vi "Assert Not Error 1097.vi"(8 "error in (no error)":errorcluster, 11 "actual value":errorcluster) -> (0 "error out":errorcluster)   [LabVIEW 2013, in "libssh2_tests.lvlib"]
uses:
  libssh2_tests.lvlib
  <vilib>/Utility/error.llb/DialogType.ctl
  <vilib>/addons/_JKI Toolkits/Caraya/classes/Assert/Assert Not Error.vi
  <vilib>/addons/_JKI Toolkits/Caraya/classes/Assert/Assert.lvclass
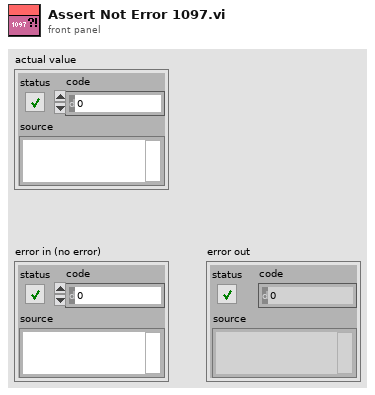
[diagram p1: front panel]
types:
  T1 = typedef "DialogType.ctl" = u16
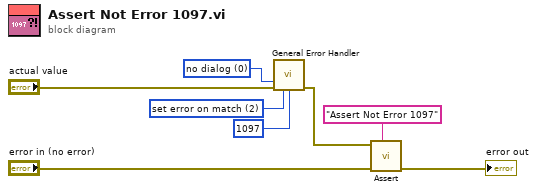
[diagram p0: block diagram]
diagram:
  w2 = T1 0 items=["no dialog", "OK message", "continue or stop message", "OK message + warnings", "continue/stop + warnings"] ("type of dialog (OK msg:1)")
  w7 = 2 items=["no exception", "cancel error on match", "set error on match"] ("[exception action] (none:0)")
  n1 = call <vilib>:"General Error Handler.vi"("type of dialog (OK msg:1)"=w2, "error in (no error)"="actual value", "[exception action] (none:0)"=w7, "[exception code]"=1097) -> ("error out"=w8:errorcluster)  [unwired: 7 in, 4 out]
  n2 = call-poly <vilib>:"Assert.vi"("Label"="Assert Not Error 1097", "error in (no error)"="error in (no error)", "Not Error?"=w8) -> ("error out"=→"error out":errorcluster)  [unwired: 7 in, 1 out]
